vi "FOCUS_V42.vi"(9 "X-pixels":sgl=256.0, 11 "Run":bool) -> (0 "Retrace pixels":sgl, 10 "Pixel Clock (Hz)":sgl)   [LabVIEW 2010] (continued)
                n476 = Add(x=w2193, y="x jog") -> (x+y=w2188:dbl[])
                n477 = And(x=w2107, y=TRUE ("XScale")) -> (x .and. y?=w2106:bool)
                n478 = Delete From Array(array=w2144, length=w2139, index=0) -> (deleted portion=w2142:dbl[], array with subset deleted=w2141:dbl[])
                n479 = Build Array (concatenate)(w2141, w2142) -> (w2111:dbl[])
                n480 = case shown="False" w2109 {
                  tunnel: w2188 -> [w2215 w2219]
                  tunnel: w2184 -> [w2214 w2218]
                  tunnel: [w2213 w2216] -> w2174
                  tunnel: w2111 -> [w2207 w2217]
                  frame False {
                    n481 = local read "Position piezo [µm]"() -> (w2211:sgl)
                    n482 = Multiply(x=sgl 40.0 ("y"), y=w2207) -> (x*y=w2208:dbl[])
                    n483 = Subtract(x=w2208, y=w2211) -> (x-y=w2206:dbl[])
                    n484 = local read "scattering length [µm]"() -> (w2209:sgl)
                    n485 = Divide(x=w2206, y=w2209) -> (x/y=w2205:dbl[])
                    n486 = local read "Intensity"() -> (w2212:sgl)
                    n487 = Exponential(1:w2205) -> (0:w2204:dbl[])
                    n488 = Multiply(x=w2204, y=w2212) -> (x*y=w2203:dbl[])
                    n489 = Build Array(w2215, w2214, w2207, w2203) -> (w2213:dbl[][])
                  }
                  frame True {
                    n490 = Build Array(w2219, w2218, w2217) -> (w2216:dbl[][])
                  }
                }
                n491 = case shown="True" w2109 {
                  tunnel: w2189 -> [_ w2262]
                  tunnel: [w2253 w2255] -> w2187
                  tunnel: [w2254 w2256] -> w2186
                  tunnel: w2174 -> [w2254 w2257]
                  frame False {
                    n492 = local read "total pixels in frame"() -> (w2253:sgl)
                  }
                  frame True {
                    n493 = local read "Scan Block Length"() -> (w2261:sgl)
                    n494 = Multiply(x=w2261, y=w2262) -> (x*y=w2260:sgl)
                    n495 = Multiply(x=w2260, y=1.0) -> (x*y=w2255:dbl)
                    n496 = Initialize Array(0.0 ("element"), 2 ("dimension size"), w2255) -> ()  [unwired: 1 out]
                    n497 = Array Subset(array=w2257, length (col)=w2255) -> (w2256:dbl[][])  [unwired: 3 in]
                  }
                }
                "y scan signals" <- w2168
                "x scan signals" <- w2169
              }
              frame 1 {
                n498 = local read "[µm] per pixel at zoom 1"() -> (w2304:sgl)
                n499 = local read "Y-lines"() -> (w2303:sgl)
                n500 = local read "Rotation z"() -> (w2279:sgl)
                n501 = local read "On?"() -> (w2280:bool)
                n502 = local read "Scanner dead time"() -> (w2296:sgl)
                n503 = case shown="False" w2280 {
                  tunnel: w2279 -> [_ w2419]
                  tunnel: [sgl 0.0 ("Rotation z") w2419] -> w2278
                  frame False {
                  }
                  frame True {
                  }
                }
                n504 = Divide(x=w2278, y=360.0) -> (x/y=w2350:dbl)
                n505 = Multiply(x=w2350, y=6.283185307179586) -> (x*y=w2348:dbl)
                n506 = Build Array(w2354, w2353, w2352) -> (w2334:dbl[][])
                n507 = Divide(x=w2296, y=w2291) -> (x/y=w2298:sgl)
                n508 = Sine(x=w2348) -> (sin(x)=w2307:dbl)
                n509 = Cosine(x=w2348) -> (cos(x)=w2347:dbl)
                n510 = Multiply(x=w2304, y=w2303) -> (x*y=w2301:sgl)
                n511 = Add(x=sgl 2.0, y=w2298) -> (x+y=w2297:sgl)
                n512 = Negate(x=w2307) -> (-x=w2346:dbl)
                n513 = Array Subset(array=w2334, length (row)=1 ("length")) -> (w2337:dbl[][])  [unwired: 3 in]
                n514 = Array Subset(array=w2334, index (row)=1 ("index")) -> (w2341:dbl[][])  [unwired: 3 in]
                n515 = local read "Zoom"() -> (w2308:sgl)
                n516 = Build Array(w2307, w2347) -> (w2343:dbl[])
                n517 = Build Array(w2347, w2346) -> (w2344:dbl[])
                n518 = local read "total y pixels"() -> (w2293:sgl)
                n519 = Round To Nearest(number=w2297) -> (nearest integer value=w2295:sgl)
                n520 = Build Array(w2344, w2343) -> (w2342:dbl[][])
                n521 = local read "Rotation"() -> (w2358:sgl)
                n522 = call-poly <vilib>:"A x B.vi"("B"=w2341, "A"=w2342) -> ("A x B"=w2335:T15)  [unwired: 1 out]
                n523 = local read "Position piezo [µm]"() -> (w2306:sgl)
                n524 = Divide(x=w2301, y=w2308) -> (x/y=w2312:sgl)
                n525 = local read "x-step (um)"() -> (w2285:sgl)
                n526 = local read "y-step (um)"() -> (w2286:sgl)
                n527 = local read "z-step (um)"() -> (w2300:sgl)
                n528 = local read "total x pixels"() -> (w2294:sgl)
                n529 = Divide(x=w2312, y=sgl 40.0) -> (x/y=w2318:sgl)
                n530 = Multiply(x=w2358, y=-1.0) -> (x*y=w2361:dbl)
                n531 = Index Array(array=w2335, index (row)=0 ("disabled index (col)")) -> (element=w2336:dbl[])  [unwired: 1 in]
                n532 = Index Array(array=w2335, index (row)=1 ("disabled index (col)")) -> (element=w2309:dbl[])  [unwired: 1 in]
                n533 = Array Max & Min(array=w2309) -> (max value=w2310:dbl, min value=w2315:dbl)  [unwired: 2 out]
                n534 = Subtract(x=w2310, y=w2315) -> (x-y=w2317:dbl)
                n535 = local read "Mode selector"() -> (w2272:u16)
                n536 = Equal To 0?(x=w2317) -> (x = 0?=w2320:bool)
                n537 = Subtract(x=w2309, y=w2315) -> (x-y=w2321:dbl[])
                n538 = Subtract(x=w2361, y=360.0) -> (x-y=w2359:dbl)
                n539 = Multiply(x=w2318, y=w2307) -> (x*y=w2319:dbl)
                n540 = Divide(x=w2359, y=360.0) -> (x/y=w2367:dbl)
                n541 = Build Array (concatenate)(w2337, w2336) -> (w2333:dbl[][])
                n542 = Equal To 0?(x=w2285) -> (x = 0?=w2284:bool)
                n543 = Equal To 0?(x=w2286) -> (x = 0?=w2283:bool)
                n544 = Equal To 0?(x=w2300) -> (x = 0?=w2282:bool)
                n545 = Divide(x=w2306, y=sgl 40.0) -> (x/y=w2302:sgl)
                n546 = case shown="False" w2320 {
                  tunnel: [w2447 w2448] -> w2316
                  tunnel: w2317 -> [w2446 _]
                  tunnel: w2319 -> [w2444 _]
                  tunnel: w2302 -> [w2442 w2450]
                  tunnel: w2321 -> [w2436 w2449]
                  frame False {
                    n547 = Divide(x=w2436, y=w2446) -> (x/y=w2445:dbl[])
                    n548 = Multiply(x=w2445, y=w2444) -> (x*y=w2443:dbl[])
                    n549 = Add(x=w2443, y=w2442) -> (x+y=w2435:dbl[])
                    n550 = Array Max & Min(array=w2435) -> (max value=w2441:dbl, min value=w2438:dbl)  [unwired: 2 out]
                    n551 = Subtract(x=w2441, y=w2438) -> (x-y=w2440:dbl)
                    n552 = Divide(x=w2440, y=2.0) -> (x/y=w2437:dbl)
                    n553 = Subtract(x=w2435, y=w2437) -> (x-y=w2447:dbl[])
                  }
                  frame True {
                    n554 = Add(x=w2449, y=w2450) -> (x+y=w2448:dbl[])
                  }
                }
                n555 = Multiply(x=w2367, y=6.283185307179586) -> (x*y=w2369:dbl)
                n556 = Compound Arithmetic op=AND(w2284, w2283, w2282) -> (w2281:bool)
                n557 = Equal?(x=w2272, y=u16 4) -> (x = y?=w2265:bool)
                n558 = Sine(x=w2369) -> (sin(x)=w2373:dbl)
                n559 = Cosine(x=w2369) -> (cos(x)=w2374:dbl)
                n560 = case shown="False" w2281 {
                  tunnel: [w2427 w2434] -> w2292
                  tunnel: w2295 -> [w2422 w2430]
                  frame True {
                    w2426 = 10178 items=["Finite Samples"=10178, "Continuous Samples"=10123, "Hardware Timed Single Point"=12522] ("sample mode")
                    n561 = local read "total pixels in frame"() -> (w2424:sgl)
                    n562 = local read "Number of frames"() -> (w2423:sgl)
                    n563 = local read "Averaging"() -> (w2425:u16)
                    n564 = Compound Arithmetic op=MULTIPLY(w2425, w2423, w2424) -> (w2421:sgl)
                    n565 = Add(x=w2421, y=w2422) -> (x+y=w2420:sgl)
                    n566 = Bundle(w2420, "sample mode"=w2426) -> (w2427:cluster{sgl, "sample mode":i32})  [unwired: 1 in]
                  }
                  frame False {
                    w2433 = 10178 items=["Finite Samples"=10178, "Continuous Samples"=10123, "Hardware Timed Single Point"=12522] ("sample mode")
                    n567 = local read "total pixels in frame"() -> (w2431:sgl)
                    n568 = local read "Averaging"() -> (w2432:u16)
                    n569 = Compound Arithmetic op=MULTIPLY(w2432, w2431) -> (w2429:sgl)
                    n570 = Add(x=w2429, y=w2430) -> (x+y=w2428:sgl)
                    n571 = Bundle(w2428, "sample mode"=w2433) -> (w2434:cluster{sgl, "sample mode":i32})  [unwired: 1 in]
                  }
                }
                n572 = Negate(x=w2373) -> (-x=w2370:dbl)
                n573 = local read "FocusModeSelector"() -> (w2276:bool)
                n574 = Build Array(w2374, w2370) -> (w2371:dbl[])
                n575 = Build Array(w2373, w2374) -> (w2372:dbl[])
                n576 = Build Array(w2371, w2372) -> (w2357:dbl[][])
                n577 = call-poly <vilib>:"A x B.vi"("B"=w2333, "A"=w2357) -> ("A x B"=w2332:T15)  [unwired: 1 out]
                n578 = In Range and Coerce(upper limit=0.0 ("element"), x=w2316, lower limit=10.0 ("element")) -> (coerced(x)=w2329:dbl[])  [unwired: 1 out]
                n579 = Divide(x=w2332, y=w2308) -> (x/y=w2331:T15)
                n580 = Array Size(array=w2329) -> (size(s)=w2328:i32)
                n581 = local read "x jog"() -> (w2289:sgl)
                n582 = local read "y jog"() -> (w2288:sgl)
                n583 = case shown="True" w2276 {
                  tunnel: w2267 -> [w2409 w2417]
                  tunnel: [w2408 w2416] -> w2266
                  tunnel: w2268 -> [w2407 w2415]
                  frame True {
                    n584 = Concatenate Strings(w2407, tag "/ao0," ("physical channels"), w2407, tag "/ao1," ("physical channels"), w2407, tag "/ao2" ("physical channels")) -> (w2404:string)
                    n585 = Type Cast(type=w2409, x=w2404) -> (*(type *) &x=w2408:tag)
                  }
                  frame False {
                    n586 = Concatenate Strings(w2415, tag "/ao0," ("physical channels"), w2415, tag "/ao1," ("physical channels"), w2415, tag "/ao2," ("physical channels"), w2415, tag "/ao3" ("physical channels")) -> (w2412:string)
                    n587 = Type Cast(type=w2417, x=w2412) -> (*(type *) &x=w2416:tag)
                  }
                }
                n588 = case shown="True" w2265 {
                  tunnel: w2267 -> [w2380 _]
                  tunnel: [w2379 w2381] -> w2264
                  tunnel: w2268 -> [w2378 _]
                  tunnel: w2266 -> [_ w2381]
                  frame True {
                    n589 = Concatenate Strings(w2378, tag "/ao0," ("physical channels"), w2378, tag "/ao1" ("physical channels")) -> (w2375:string)
                    n590 = Type Cast(type=w2380, x=w2375) -> (*(type *) &x=w2379:tag)
                  }
                  frame False {
                  }
                }
                n591 = Index Array(array=w2331, index (row)=0 ("disabled index (col)")) -> (element=w2365:dbl[])  [unwired: 1 in]
                n592 = Index Array(array=w2331, index (row)=1 ("disabled index (col)")) -> (element=w2364:dbl[])  [unwired: 1 in]
                n593 = Multiply(x=w2328, y=15) -> (x*y=w2323:i32)
                n594 = local read "total pixels in frame"() -> (w2290:sgl)
                n595 = Divide(x=w2323, y=360.0) -> (x/y=w2324:dbl)
                n596 = Add(x=w2364, y=w2288) -> (x+y=w2273:dbl[])
                n597 = Add(x=w2365, y=w2289) -> (x+y=w2274:dbl[])
                n598 = Not(x=w2276) -> (.not. x?=w2275:bool)
                n599 = Delete From Array(array=w2329, length=w2324, index=0) -> (deleted portion=w2327:dbl[], array with subset deleted=w2326:dbl[])
                n600 = Build Array (concatenate)(w2326, w2327) -> (w2277:dbl[])
                n601 = case shown="False" w2276 {
                  tunnel: w2274 -> [w2398 w2402]
                  tunnel: w2273 -> [w2397 w2401]
                  tunnel: [w2396 w2399] -> w2270
                  tunnel: w2277 -> [w2393 w2400]
                  frame False {
                    n602 = local read "Position piezo [µm]"() -> (w2388:sgl)
                    n603 = Multiply(x=sgl 40.0 ("y"), y=w2393) -> (x*y=w2394:dbl[])
                    n604 = Subtract(x=w2394, y=w2388) -> (x-y=w2392:dbl[])
                    n605 = local read "scattering length [µm]"() -> (w2387:sgl)
                    n606 = Divide(x=w2392, y=w2387) -> (x/y=w2391:dbl[])
                    n607 = Exponential(1:w2391) -> (0:w2390:dbl[])
                    n608 = local read "Intensity"() -> (w2386:sgl)
                    n609 = Multiply(x=w2390, y=w2386) -> (x*y=w2389:dbl[])
                    n610 = Build Array(w2398, w2397, w2393, w2389) -> (w2396:dbl[][])
                  }
                  frame True {
                    n611 = Build Array(w2402, w2401, w2400) -> (w2399:dbl[][])
                  }
                }
                n612 = case shown="False" w2265 {
                  tunnel: w2274 -> [_ w2385]
                  tunnel: w2273 -> [_ w2384]
                  tunnel: w2270 -> [w2382 _]
                  tunnel: [w2382 w2383] -> w2269
                  frame False {
                  }
                  frame True {
                    n613 = Build Array(w2385, w2384) -> (w2383:dbl[][])
                  }
                }
              }
              frame 2 {
                w2465 = 10123 items=["Finite Samples"=10178, "Continuous Samples"=10123, "Hardware Timed Single Point"=12522] ("sample mode")
                n614 = local read "[µm] per pixel at zoom 1"() -> (w2472:sgl)
                n615 = local read "Y-lines"() -> (w2471:sgl)
                n616 = local read "Rotation z"() -> (w2452:sgl)
                n617 = local read "On?"() -> (w2453:bool)
                n618 = case shown="False" w2453 {
                  tunnel: w2452 -> [_ w2552]
                  tunnel: [sgl 0.0 ("Rotation z") w2552] -> w2451
                  frame False {
                  }
                  frame True {
                  }
                }
                n619 = Divide(x=w2451, y=360.0) -> (x/y=w2519:dbl)
                n620 = case shown="False" "Linescan mode" {
                  tunnel: w2458 -> [w2554 _]
                  tunnel: [w2554 w2557] -> w2457
                  tunnel: [w2553 w2558] -> w2456
                  tunnel: w2455 -> [_ w2558]
                  frame False {
                    n621 = Array Size(array=w2554) -> (size(s)=w2555:i32)
                    n622 = Initialize Array(0.0 ("element"), w2555) -> (w2553:dbl[])
                  }
                  frame True {
                    n623 = Array Size(array=w2558) -> (size(s)=w2559:i32)
                    n624 = Initialize Array(0.0 ("element"), w2559) -> (w2557:dbl[])
                  }
                }
                n625 = Multiply(x=w2519, y=6.283185307179586) -> (x*y=w2517:dbl)
                n626 = Build Array(w2457, w2456, w2521) -> (w2503:dbl[][])
                n627 = Sine(x=w2517) -> (sin(x)=w2475:dbl)
                n628 = Cosine(x=w2517) -> (cos(x)=w2516:dbl)
                n629 = Multiply(x=w2472, y=w2471) -> (x*y=w2469:sgl)
                n630 = Negate(x=w2475) -> (-x=w2515:dbl)
                n631 = Array Subset(array=w2503, length (row)=1 ("length")) -> (w2506:dbl[][])  [unwired: 3 in]
                n632 = Array Subset(array=w2503, index (row)=1 ("index")) -> (w2510:dbl[][])  [unwired: 3 in]
                n633 = local read "Zoom"() -> (w2477:sgl)
                n634 = Build Array(w2475, w2516) -> (w2512:dbl[])
                n635 = Build Array(w2516, w2515) -> (w2513:dbl[])
                n636 = local read "total y pixels"() -> (w2463:sgl)
                n637 = Build Array(w2513, w2512) -> (w2511:dbl[][])
                n638 = local read "Rotation"() -> (w2532:sgl)
                n639 = local read "total x pixels"() -> (w2462:sgl)
                n640 = call-poly <vilib>:"A x B.vi"("B"=w2510, "A"=w2511) -> ("A x B"=w2504:T15)  [unwired: 1 out]
                n641 = local read "Position piezo [µm]"() -> (w2474:sgl)
                n642 = Divide(x=w2469, y=w2477) -> (x/y=w2481:sgl)
                n643 = Divide(x=w2481, y=sgl 40.0) -> (x/y=w2487:sgl)
                n644 = Multiply(x=w2532, y=-1.0) -> (x*y=w2535:dbl)
                n645 = Index Array(array=w2504, index (row)=0 ("disabled index (col)")) -> (element=w2505:dbl[])  [unwired: 1 in]
                n646 = Index Array(array=w2504, index (row)=1 ("disabled index (col)")) -> (element=w2478:dbl[])  [unwired: 1 in]
                n647 = Array Max & Min(array=w2478) -> (max value=w2479:dbl, min value=w2484:dbl)  [unwired: 2 out]
                n648 = Subtract(x=w2479, y=w2484) -> (x-y=w2486:dbl)
                n649 = Equal To 0?(x=w2486) -> (x = 0?=w2489:bool)
                n650 = Subtract(x=w2478, y=w2484) -> (x-y=w2490:dbl[])
                n651 = Subtract(x=w2535, y=360.0) -> (x-y=w2533:dbl)
                n652 = Multiply(x=w2487, y=w2475) -> (x*y=w2488:dbl)
                n653 = Divide(x=w2533, y=360.0) -> (x/y=w2543:dbl)
                n654 = Build Array (concatenate)(w2506, w2505) -> (w2502:dbl[][])
                n655 = Divide(x=w2474, y=sgl 40.0) -> (x/y=w2470:sgl)
                n656 = case shown="False" w2489 {
                  tunnel: [w2573 w2574] -> w2485
                  tunnel: w2486 -> [w2572 _]
                  tunnel: w2488 -> [w2570 _]
                  tunnel: w2470 -> [w2568 w2576]
                  tunnel: w2490 -> [w2562 w2575]
                  frame False {
                    n657 = Divide(x=w2562, y=w2572) -> (x/y=w2571:dbl[])
                    n658 = Multiply(x=w2571, y=w2570) -> (x*y=w2569:dbl[])
                    n659 = Add(x=w2569, y=w2568) -> (x+y=w2561:dbl[])
                    n660 = Array Max & Min(array=w2561) -> (max value=w2567:dbl, min value=w2564:dbl)  [unwired: 2 out]
                    n661 = Subtract(x=w2567, y=w2564) -> (x-y=w2566:dbl)
                    n662 = Divide(x=w2566, y=2.0) -> (x/y=w2563:dbl)
                    n663 = Subtract(x=w2561, y=w2563) -> (x-y=w2573:dbl[])
                  }
                  frame True {
                    n664 = Add(x=w2575, y=w2576) -> (x+y=w2574:dbl[])
                  }
                }
                n665 = Multiply(x=w2543, y=6.283185307179586) -> (x*y=w2545:dbl)
                n666 = Sine(x=w2545) -> (sin(x)=w2549:dbl)
                n667 = Cosine(x=w2545) -> (cos(x)=w2550:dbl)
                n668 = Negate(x=w2549) -> (-x=w2546:dbl)
                n669 = Build Array(w2550, w2546) -> (w2547:dbl[])
                n670 = Build Array(w2549, w2550) -> (w2548:dbl[])
                n671 = Bundle("sample mode"=w2465, "sample mode"=w2465) -> (w2461:cluster{"sample mode":i32, "sample mode":i32})  [unwired: 1 in]
                n672 = Build Array(w2547, w2548) -> (w2531:dbl[][])
                n673 = call-poly <vilib>:"A x B.vi"("B"=w2502, "A"=w2531) -> ("A x B"=w2501:T15)  [unwired: 1 out]
                n674 = In Range and Coerce(upper limit=0.0 ("element"), x=w2485, lower limit=10.0 ("element")) -> (coerced(x)=w2498:dbl[])  [unwired: 1 out]
                n675 = Divide(x=w2501, y=w2477) -> (x/y=w2500:T15)
                n676 = Array Size(array=w2498) -> (size(s)=w2497:i32)
                n677 = local read "x jog"() -> (w2467:sgl)
                n678 = local read "y jog"() -> (w2466:sgl)
                n679 = Index Array(array=w2500, index (row)=0 ("disabled index (col)")) -> (element=w2541:dbl[])  [unwired: 1 in]
                n680 = Index Array(array=w2500, index (row)=1 ("disabled index (col)")) -> (element=w2540:dbl[])  [unwired: 1 in]
                n681 = Multiply(x=w2497, y=15) -> (x*y=w2492:i32)
                n682 = Divide(x=w2492, y=360.0) -> (x/y=w2493:dbl)
                n683 = Add(x=w2540, y=w2466) -> (x+y=w2537:dbl[])
                n684 = Multiply(x=w2462, y=sgl 1.0) -> (x*y=w2460:sgl)
                n685 = Add(x=w2541, y=w2467) -> (x+y=w2539:dbl[])
                n686 = Delete From Array(array=w2498, length=w2493, index=0) -> (deleted portion=w2496:dbl[], array with subset deleted=w2495:dbl[])
                n687 = Concatenate Strings(w2527, tag "/ao0," ("physical channels"), w2527, tag "/ao1," ("physical channels"), w2527, tag "/ao2" ("physical channels")) -> (w2523:string)
                n688 = Build Array (concatenate)(w2495, w2496) -> (w2476:dbl[])
                n689 = Build Array(w2539, w2537, w2476) -> (w2468:dbl[][])
                n690 = Type Cast(type=w2528, x=w2523) -> (*(type *) &x=w2526:tag)
              }
              frame 3 {
                w2581 = 10123 items=["Finite Samples"=10178, "Continuous Samples"=10123, "Hardware Timed Single Point"=12522] ("sample mode")
                n691 = case shown="True" w2591 {
                  tunnel: w2595 -> [_ _]
                  tunnel: [w2599 w2618] -> w2590
                  tunnel: [w2601 w2636] -> w2594
                  tunnel: [w2600 w2613] -> w2593
                  tunnel: [w2600 w2613] -> w2592
                  tunnel: w2579 -> [_ w2610]
                  tunnel: w2578 -> [_ w2606]
                  frame False {
                    n692 = local read "Y-lines FreeLine"() -> (w2601:sgl)
                    n693 = local read "X-pixels FreeLine"() -> (w2600:sgl)
                    n694 = local read "y scan signals"() -> (w2596:dbl[])
                    n695 = Array Max & Min(array=w2596) -> (max value=w2598:dbl, min value=w2597:dbl)  [unwired: 2 out]
                    n696 = property on="XY Graph 1" class="XYGraph (strict)"("X Scale.Range:Maximum"=w2598, "X Scale.Range:Minimum"=w2597, "Y Scale.Range:Maximum"=w2598, "Y Scale.Range:Minimum"=w2597) -> ()  [unwired: 2 in, 2 out]
                    n697 = property on="XY Graph 2" class="XYGraph (strict)"("X Scale.Range:Maximum"=w2598, "X Scale.Range:Minimum"=w2597, "Y Scale.Range:Maximum"=w2598, "Y Scale.Range:Minimum"=w2597) -> ()  [unwired: 2 in, 2 out]
                    n698 = local read "ScanLineFreeLine"() -> (w2599:sgl[][])
                  }
                  frame True {
                    w2654 = 1 ("length")
                    # "Rotation"
                    n699 = local read "Scan Cut-Off (either end)"() -> (w2603:sgl)
                    n700 = Index Array(array=w2606, index=w2603) -> (element=w2609:dbl)
                    n701 = local read "X-pixels"() -> (w2605:sgl)
                    n702 = local read "Y-lines"() -> (w2604:sgl)
                    n703 = property on="XY Graph 2" class="XYGraph (strict)"("Visible"=TRUE) -> ()  [unwired: 2 in, 2 out]
                    n704 = property on="XY Graph 1" class="XYGraph (strict)"("Visible"=TRUE) -> ()  [unwired: 2 in, 2 out]
                    n705 = Divide(x=w2605, y=w2604) -> (x/y=w2608:sgl)
                    n706 = property on="Image 2" class="IntGraph (strict)"() -> ("Color Table"=w2644:u32[])  [unwired: 2 in, 2 out]
                    n707 = Divide(x=w2609, y=w2608) -> (x/y=w2607:dbl)
                    n708 = Absolute Value(x=w2607) -> (abs(x)=w2602:dbl)
                    n709 = local read "Image 2"() -> (w2669:u8[][])
                    n710 = local read "Image 1"() -> (w2668:u8[][])
                    n711 = local read "X-pixels"() -> (w2633:sgl)
                    n712 = local read "Y-lines"() -> (w2632:sgl)
                    n713 = call "FreeLine2D.vi"("Color Table"=w2644, "data channel 2"=w2669, "X-pixels"=w2633, "Y-lines"=w2632, "data channel"=w2668) -> ("user defined lines"=w2636:i16, "PointsCoordinates"=w2638:i32[][], "pixel x"=w2635:dbl[], "pixel y"=w2634:dbl[], "number of pixels"=w2613:dbl, "Pixel Clock (Hz)"=w2612:dbl)
                    "X-pixels FreeLine" <- w2613
                    "Pixel Clock (Hz) FreeLine" <- w2612
                    n714 = local write "Y-lines FreeLine"(w2636) -> ()
                    n715 = Array Max & Min(array=w2610) -> (max value=w2617:dbl, min value=w2616:dbl)  [unwired: 2 out]
                    n716 = call "CalcxyscansignalsudlFOCUS.vi"("Y-Lines"=w2632, "X Pixels"=w2633, "MaxValuey"=w2602, "MaxValuex"=w2602, "pixel y"=w2634, "pixel x"=w2635) -> ("Signal y"=w2630:dbl[], "Signal x"=w2631:dbl[])
                    n717 = Index Array(array=w2638, index (col)=0 ("disabled index (col)")) -> (element=w2642:i32[])  [unwired: 1 in]
                    n718 = Index Array(array=w2638, index (col)=1 ("disabled index (col)")) -> (element=w2641:i32[])  [unwired: 1 in]
                    n719 = local write "new FreeLine?"(FALSE ("new udl?")) -> ()
                    n720 = Bundle("PointsCoordinates"=w2642, "PointsCoordinates"=w2641) -> (w2637:T16)  [unwired: 1 in]
                    n721 = local read "Rotation"() -> (w2626:sgl)
                    n722 = property on="XY Graph 1" class="XYGraph (strict)"("X Scale.Range:Maximum"=w2617, "X Scale.Range:Minimum"=w2616, "Y Scale.Range:Maximum"=w2617, "Y Scale.Range:Minimum"=w2616) -> ()  [unwired: 2 in, 2 out]
                    n723 = Build Array(w2631, w2630) -> (w2623:dbl[][])
                    n724 = Multiply(x=w2626, y=-1.0) -> (x*y=w2628:dbl)
                    n725 = local write "Histogram1"(w2637) -> ()
                    n726 = local write "Histogram2"(w2637) -> ()
                    n727 = Subtract(x=w2628, y=360.0) -> (x-y=w2625:dbl)
                    n728 = local read "Zoom"() -> (w2651:sgl)
                    n729 = Divide(x=w2625, y=360.0) -> (x/y=w2677:dbl)
                    n730 = property on="XY Graph 2" class="XYGraph (strict)"("X Scale.Range:Maximum"=w2617, "X Scale.Range:Minimum"=w2616, "Y Scale.Range:Maximum"=w2617, "Y Scale.Range:Minimum"=w2616) -> ()  [unwired: 2 in, 2 out]
                    n731 = Multiply(x=w2677, y=6.283185307179586) -> (x*y=w2675:dbl)
                    n732 = Divide(x=w2623, y=w2651) -> (x/y=w2622:dbl[][])
                    n733 = Reciprocal(x=w2612) -> (1/x=w2615:dbl)
                    n734 = property on="XY Graph 3" class="XYGraph (strict)"("X Scale.Range:Maximum"=w2617, "X Scale.Range:Minimum"=w2616, "Y Scale.Range:Maximum"=w2617, "Y Scale.Range:Minimum"=w2616) -> ()  [unwired: 2 in, 2 out]
                    n735 = Sine(x=w2675) -> (sin(x)=w2671:dbl)
                    n736 = Cosine(x=w2675) -> (cos(x)=w2670:dbl)
                    n737 = Negate(x=w2671) -> (-x=w2674:dbl)
                    n738 = Multiply(x=w2615, y=sgl 1000000.0) -> (x*y=w2611:dbl)
                    n739 = Array Subset(array=w2631, index=0, length=1) -> (w2661:dbl[])
                    n740 = Array Subset(array=w2630, index=0, length=1) -> (w2660:dbl[])
                    n741 = local write "pixel dwell time [us] FreeLine"(w2611) -> ()
                    n742 = Build Array(w2670, w2674) -> (w2673:dbl[])
                    n743 = Build Array(w2671, w2670) -> (w2672:dbl[])
                    n744 = property on="XY Graph 4" class="XYGraph (strict)"("X Scale.Range:Maximum"=w2617, "X Scale.Range:Minimum"=w2616, "Y Scale.Range:Maximum"=w2617, "Y Scale.Range:Minimum"=w2616) -> ()  [unwired: 2 in, 2 out]
                    n745 = Bundle("Signal x"=w2631, "Signal y"=w2630) -> (w2659:cluster{"Signal x":dbl[], "Signal y":dbl[]})  [unwired: 1 in]
                    n746 = Bundle(w2661, w2660) -> (w2658:cluster{dbl[], dbl[]})  [unwired: 1 in]
                    n747 = Build Array(w2673, w2672) -> (w2624:dbl[][])
                    n748 = Decrement(x=w2613) -> (x-1=w2653:dbl)
                    n749 = Array Subset(array=w2631, index=w2653, length=w2654) -> (w2655:dbl[])
                    n750 = Array Subset(array=w2630, index=w2653, length=w2654) -> (w2656:dbl[])
                    n751 = call-poly <vilib>:"A x B.vi"("B"=w2622, "A"=w2624) -> ("A x B"=w2621:T15)  [unwired: 1 out]
                    n752 = Bundle(w2655, w2656) -> (w2652:cluster{dbl[], dbl[]})  [unwired: 1 in]
                    n753 = local read "x jog"() -> (w2645:sgl)
                    n754 = Index Array(array=w2621, index (row)=0 ("disabled index (col)")) -> (element=w2650:dbl[])  [unwired: 1 in]
                    n755 = Index Array(array=w2621, index (row)=1 ("disabled index (col)")) -> (element=w2649:dbl[])  [unwired: 1 in]
                    n756 = Build Array(w2659, w2658, w2652) -> (→"XY Graph 1" →"XY Graph 2":cluster{"Signal x":dbl[], "Signal y":dbl[]}[])
                    n757 = local read "y jog"() -> (w2646:sgl)
                    n758 = Add(x=w2649, y=w2646) -> (x+y=w2647:dbl[])
                    n759 = Add(x=w2650, y=w2645) -> (x+y=w2648:dbl[])
                    n760 = Build Array(w2648, w2647) -> (w2618:dbl[][])
                    "ScanLineFreeLine" <- w2618
                  }
                }
                n761 = Bundle("sample mode"=w2581, "sample mode"=w2581) -> (w2580:cluster{"sample mode":i32, "sample mode":i32})  [unwired: 1 in]
                n762 = local write "XScale"(TRUE ("XScale")) -> ()
                n763 = Concatenate Strings(w2585, tag "/ao0," ("physical channels"), w2585, tag "/ao1" ("physical channels")) -> (w2587:string)
                n764 = Type Cast(type=w2584, x=w2587) -> (*(type *) &x=w2583:tag)
              }
              frame 4 {
                w2685 = 10123 items=["Finite Samples"=10178, "Continuous Samples"=10123, "Hardware Timed Single Point"=12522] ("sample mode")
                n765 = case shown="True" w2694 {
                  tunnel: [w2730 w2782] -> w2700
                  tunnel: [w2729 w2745] -> w2696
                  tunnel: w2699 -> [_ _]
                  tunnel: [w2705 w2754] -> w2698
                  tunnel: [w2729 w2745] -> w2697
                  tunnel: w2683 -> [_ w2748]
                  tunnel: w2682 -> [_ w2747]
                  tunnel: w2681 -> [_ w2738]
                  tunnel: w2680 -> [_ w2737]
                  frame False {
                    n766 = local read "Zsin3D"() -> (w2713:sgl[])
                    n767 = local read "Amplitude Factor"() -> (w2711:sgl)
                    n768 = local read "y scan signals"() -> (w2719:dbl[])
                    n769 = Array Size(array=w2713) -> (size(s)=w2718:i32)
                    n770 = Add Array Elements(numeric array=w2713) -> (sum=w2717:sgl)
                    n771 = Divide(x=w2717, y=w2718) -> (x/y=w2714:sgl)
                    n772 = Subtract(x=w2713, y=w2714) -> (x-y=w2716:sgl[])
                    n773 = Multiply(x=w2716, y=w2711) -> (x*y=w2715:sgl[])
                    n774 = local read "phase shift [°]"() -> (w2722:sgl)
                    n775 = Array Max & Min(array=w2719) -> (max value=w2721:dbl, min value=w2720:dbl)  [unwired: 2 out]
                    n776 = Add(x=w2715, y=w2714) -> (x+y=w2712:sgl[])
                    n777 = local read "Y-lines FreeLine"() -> (w2730:sgl)
                    n778 = local read "X-pixels FreeLine"() -> (w2729:sgl)
                    n779 = property on="XY Graph 1" class="XYGraph (strict)"("X Scale.Range:Maximum"=w2721, "X Scale.Range:Minimum"=w2720, "Y Scale.Range:Maximum"=w2721, "Y Scale.Range:Minimum"=w2720) -> ()  [unwired: 2 in, 2 out]
                    n780 = Array Size(array=w2712) -> (size(s)=w2706:i32)
                    n781 = Multiply(x=w2706, y=w2722) -> (x*y=w2727:sgl)
                    n782 = Divide(x=w2727, y=360.0) -> (x/y=w2726:dbl)
                    n783 = property on="XY Graph 2" class="XYGraph (strict)"("X Scale.Range:Maximum"=w2721, "X Scale.Range:Minimum"=w2720, "Y Scale.Range:Maximum"=w2721, "Y Scale.Range:Minimum"=w2720) -> ()  [unwired: 2 in, 2 out]
                    n784 = local read "Intensity"() -> (w2707:sgl)
                    n785 = local read "ZInt3D"() -> (w2708:sgl[])
                    n786 = Delete From Array(array=w2712, length=w2726, index=0) -> (deleted portion=w2723:sgl[], array with subset deleted=w2724:sgl[])
                    n787 = Build Array (concatenate)(w2724, w2723) -> (w2710:sgl[])
                    n788 = Multiply(x=w2708, y=w2707) -> (x*y=w2702:sgl[])
                    n789 = Initialize Array(w2707, w2706) -> ()  [unwired: 1 out]
                    n790 = property on="Histogram1" class="XYGraph (strict)"("Visible"=FALSE) -> ()  [unwired: 2 in, 2 out]
                    n791 = case shown="True" "Int Corr?" {
                      tunnel: w2702 -> [w2731 w2736]
                      tunnel: [w2731 w2735] -> w2701
                      frame False {
                      }
                      frame True {
                        n792 = local read "Image3Arrayd"() -> (w2732:u8[][])
                        n793 = call "NormalizeIntensityUDL3D.vi"("bigger"="Scale", "Image3Array"=w2732, "Pockel's cell original"=w2736, "File?"=FALSE) -> ("Pockel's cell corrected"=w2735:dbl[])
                      }
                    }
                    n794 = local read "ScanLineFreeLine"() -> (w2709:sgl[][])
                    n795 = Build Array (concatenate)(w2709, w2710, w2701) -> (w2705:dbl[][])
                  }
                  frame True {
                    w2820 = 1 ("length")
                    # "Rotation"
                    n796 = property on="Image 2" class="IntGraph (strict)"() -> ("Color Table"=w2791:u32[])  [unwired: 2 in, 2 out]
                    n797 = local read "Scan Cut-Off (either end)"() -> (w2800:sgl)
                    n798 = local write "new FreeLine?"(FALSE ("new 3D udl?")) -> ()
                    n799 = local read "pixelstoµm"() -> (w2812:sgl)
                    n800 = property on="XY Graph 2" class="XYGraph (strict)"("Visible"=TRUE) -> ()  [unwired: 2 in, 2 out]
                    n801 = property on="XY Graph 1" class="XYGraph (strict)"("Visible"=TRUE) -> ()  [unwired: 2 in, 2 out]
                    n802 = local read "Number of frames"() -> (w2816:sgl)
                    n803 = local read "X-pixels"() -> (w2802:sgl)
                    n804 = local read "Y-lines"() -> (w2801:sgl)
                    n805 = Index Array(array=w2738, index=w2800) -> (element=w2739:dbl)
                    n806 = Divide(x=w2802, y=w2801) -> (x/y=w2803:sgl)
                    n807 = local read "X-pixels"() -> (w2770:sgl)
                    n808 = local read "Y-lines"() -> (w2769:sgl)
                    n809 = Divide(x=w2739, y=w2803) -> (x/y=w2799:dbl)
                    n810 = local read "z-step (um)"() -> (w2817:sgl)
                    n811 = Absolute Value(x=w2799) -> (abs(x)=w2771:dbl)
                    n812 = local read "Zoom"() -> (w2813:sgl)
                    n813 = call "FreeLine3D.vi"("Data1"=w2748, "z step (µm)"=w2817, "Color Table"=w2791, "Y-lines"=w2769, "X-pixels"=w2770, "Data2"=w2747, "pixelstoµm"=w2812, "z planes"=w2816, "zoom"=w2813) -> ("user defined lines"=w2782:i16, "x-values [pixels]"=w2773:dbl[], "pockel's cell"=w2752:dbl[], "y-values [pixels]"=w2772:dbl[], "PointsCoordinates"=w2787:i32[][], "pixel clock [Hz]"=w2743:dbl, "z-values [µm]"=w2746:dbl[])
                    "Pixel Clock z (Hz) FreeLine" <- w2743
                    "PointsCoordinates" <- w2787
                    "ZInt3D" <- w2752
                    n814 = local write "Y-lines FreeLine"(w2782) -> ()
                    n815 = Divide(x=w2746, y=40.0) -> (x/y=w2778:dbl[])
                    "Zsin3D" <- w2778
                    n816 = Array Size(array=w2778) -> (size(s)=w2749:i32)
                    n817 = Add Array Elements(numeric array=w2778) -> (sum=w2781:dbl)
                    n818 = Divide(x=w2781, y=w2749) -> (x/y=w2776:dbl)
                    n819 = Subtract(x=w2778, y=w2776) -> (x-y=w2780:dbl[])
                    n820 = Multiply(x=w2780, y="Amplitude Factor") -> (x*y=w2777:dbl[])
                    n821 = Add(x=w2777, y=w2776) -> (x+y=w2775:dbl[])
                    n822 = Array Size(array=w2775) -> (size(s)=w2809:i32)
                    n823 = Array Size(array=w2746) -> (size(s)=w2745:i32)
                    n824 = Array Max & Min(array=w2737) -> (max value=w2790:dbl, min value=w2789:dbl)  [unwired: 2 out]
                    n825 = call "CalcxyscansignalsudlFOCUS.vi"("Y-Lines"=w2769, "X Pixels"=w2770, "MaxValuey"=w2771, "MaxValuex"=w2771, "pixel y"=w2772, "pixel x"=w2773) -> ("Signal y"=w2767:dbl[], "Signal x"=w2768:dbl[])
                    n826 = Multiply(x=w2809, y="phase shift [°]") -> (x*y=w2810:sgl)
                    n827 = Divide(x=w2810, y=360.0) -> (x/y=w2807:dbl)
                    n828 = local write "Pixel Clock (Hz) FreeLine"(w2743) -> ()
                    n829 = Delete From Array(array=w2775, length=w2807, index=0) -> (deleted portion=w2804:dbl[], array with subset deleted=w2805:dbl[])
                    n830 = Build Array(w2768, w2767) -> (w2760:dbl[][])
                    n831 = property on="XY Graph 1" class="XYGraph (strict)"("X Scale.Range:Maximum"=w2790, "X Scale.Range:Minimum"=w2789, "Y Scale.Range:Maximum"=w2790, "Y Scale.Range:Minimum"=w2789) -> ()  [unwired: 2 in, 2 out]
                    n832 = Build Array (concatenate)(w2805, w2804) -> (w2755:dbl[])
                    n833 = Index Array(array=w2787, index (col)=0 ("disabled index (col)")) -> (element=w2788:i32[])  [unwired: 1 in]
                    n834 = Index Array(array=w2787, index (col)=1 ("disabled index (col)")) -> (element=w2786:i32[])  [unwired: 1 in]
                    n835 = local read "Rotation"() -> (w2763:sgl)
                    n836 = local read "Intensity"() -> (w2751:sgl)
                    n837 = Multiply(x=w2763, y=-1.0) -> (x*y=w2765:dbl)
                    n838 = local read "Zoom"() -> (w2798:sgl)
                    n839 = property on="XY Graph 2" class="XYGraph (strict)"("X Scale.Range:Maximum"=w2790, "X Scale.Range:Minimum"=w2789, "Y Scale.Range:Maximum"=w2790, "Y Scale.Range:Minimum"=w2789) -> ()  [unwired: 2 in, 2 out]
                    n840 = Bundle("PointsCoordinates"=w2788, "PointsCoordinates"=w2786) -> (→"Histogram1" →"Histogram2":T16)  [unwired: 1 in]
                    n841 = Subtract(x=w2765, y=360.0) -> (x-y=w2762:dbl)
                    n842 = Divide(x=w2760, y=w2798) -> (x/y=w2759:dbl[][])
                    n843 = Reciprocal(x=w2743) -> (1/x=w2742:dbl)
                    n844 = Divide(x=w2762, y=360.0) -> (x/y=w2840:dbl)
                    n845 = Multiply(x=w2752, y=w2751) -> ()  [unwired: 1 out]
                    n846 = local write "X-pixels FreeLine"(w2745) -> ()
                    n847 = Multiply(x=w2840, y=6.283185307179586) -> (x*y=w2838:dbl)
                    n848 = Multiply(x=w2742, y=sgl 1000000.0) -> (x*y=→"pixel dwell time [us] FreeLine":dbl)
                    n849 = Sine(x=w2838) -> (sin(x)=w2834:dbl)
                    n850 = Cosine(x=w2838) -> (cos(x)=w2833:dbl)
                    n851 = local read "x jog"() -> (w2794:sgl)
                    n852 = Array Subset(array=w2768, index=0, length=1) -> (w2826:dbl[])
                    n853 = Array Subset(array=w2767, index=0, length=1) -> (w2825:dbl[])
                    n854 = Negate(x=w2834) -> (-x=w2837:dbl)
                    n855 = local read "y jog"() -> (w2793:sgl)
                    n856 = Bundle("Signal x"=w2768, "Signal y"=w2767) -> (w2824:cluster{"Signal x":dbl[], "Signal y":dbl[]})  [unwired: 1 in]
                    n857 = Bundle(w2826, w2825) -> (w2823:cluster{dbl[], dbl[]})  [unwired: 1 in]
                    n858 = Divide(x=w2743, y=w2745) -> (x/y=w2744:dbl)
                    n859 = Build Array(w2833, w2837) -> (w2836:dbl[])
                    n860 = Build Array(w2834, w2833) -> (w2835:dbl[])
                    n861 = Decrement(x=w2745) -> (x-1=w2819:i32)
                    n862 = local write "z frequency"(w2744) -> ()
                    n863 = Build Array(w2836, w2835) -> (w2761:dbl[][])
                    n864 = Initialize Array(w2751, w2749) -> (w2750:sgl[])
                    n865 = Array Subset(array=w2768, index=w2819, length=w2820) -> (w2821:dbl[])
                    n866 = Array Subset(array=w2767, index=w2819, length=w2820) -> (w2822:dbl[])
                    n867 = call-poly <vilib>:"A x B.vi"("B"=w2759, "A"=w2761) -> ("A x B"=w2758:T15)  [unwired: 1 out]
                    n868 = Index Array(array=w2758, index (row)=0 ("disabled index (col)")) -> (element=w2797:dbl[])  [unwired: 1 in]
                    n869 = Index Array(array=w2758, index (row)=1 ("disabled index (col)")) -> (element=w2796:dbl[])  [unwired: 1 in]
                    n870 = Add(x=w2796, y=w2793) -> (x+y=w2795:dbl[])
                    n871 = Add(x=w2797, y=w2794) -> (x+y=w2774:dbl[])
                    n872 = Build Array(w2774, w2795) -> (w2753:dbl[][])
                    n873 = local write "ScanLineFreeLine"(w2753) -> ()
                    n874 = Bundle(w2821, w2822) -> (w2818:cluster{dbl[], dbl[]})  [unwired: 1 in]
                    n875 = Build Array (concatenate)(w2753, w2755, w2750) -> (w2754:dbl[][])
                    n876 = Build Array(w2824, w2823, w2818) -> (w2814:cluster{"Signal x":dbl[], "Signal y":dbl[]}[])
                    n877 = local write "XY Graph 1"(w2814) -> ()
                    n878 = local write "XY Graph 2"(w2814) -> ()
                  }
                }
                n879 = Bundle("sample mode"=w2685, "sample mode"=w2685) -> (w2684:cluster{"sample mode":i32, "sample mode":i32})  [unwired: 1 in]
                n880 = Concatenate Strings(w2688, tag "/ao0," ("physical channels"), w2688, tag "/ao1," ("physical channels"), w2688, tag "/ao2," ("physical channels"), w2688, tag "/ao3" ("physical channels")) -> (w2690:string)
                n881 = Type Cast(type=w2687, x=w2690) -> (*(type *) &x=w2686:tag)
              }
            }
          }
          frame True {
            n882 = case shown="True" "NewScanpattern" {
              tunnel: [w2932 w2942] -> w2852
              tunnel: [w2924 w2933] -> w2850
              tunnel: [w2925 w2934] -> w2849
              tunnel: [w2930 w2939] -> w2848
              tunnel: [w2924 w2933] -> w2845
              frame False {
                n883 = local read "ParametersFScope"() -> (w2931:T7)
                n884 = local read "ScanLineFScope"() -> (w2932:sgl[][])
                n885 = Unbundle(w2931) -> ("X frequeny [Hz]"=w2926:i32, "Y frequency \n[Hz]"=w2930:i32, "frequeny Trim"=w2927:dbl, "Samples/s"=w2924:i32)  [unwired: 2 out]
                n886 = local write "Pixel Clock (Hz) FScope"(w2924) -> ()
                n887 = Divide(x=w2927, y=200.0) -> (x/y=w2928:dbl)
                n888 = Add(x=w2926, y=w2928) -> (x+y=w2925:dbl)
              }
              frame True {
                n889 = call "LissajousPatternFScope.vi"("f max Y [Hz]"="f max Y", "f min Y [Hz]"="f min Y", "f max X [Hz]"="f max X", "f min X [Hz]"="f min X") -> ("Parameters"=w2940:T7, "ScanData"=w2942:dbl[][])  [unwired: 1 out]
                "ScanLineFScope" <- w2942
                "ParametersFScope" <- w2940
                n890 = Unbundle(w2940) -> ("X frequeny [Hz]"=w2935:i32, "Y frequency \n[Hz]"=w2939:i32, "frequeny Trim"=w2936:dbl, "Samples/s"=w2933:i32)  [unwired: 2 out]
                "Pixel Clock (Hz) FScope" <- w2933
                n891 = local write "NewScanpattern"(FALSE ("NewScanpattern")) -> ()
                n892 = Divide(x=w2936, y=200.0) -> (x/y=w2938:dbl)
                n893 = Add(x=w2935, y=w2938) -> (x+y=w2934:dbl)
              }
            }
            n894 = local read "scans to read"() -> (w2847:sgl)
            n895 = Reciprocal(x=w2845) -> (1/x=w2846:dbl)
            n896 = Multiply(x=w2846, y=w2847) -> (x*y=w2844:dbl)
            n897 = Reciprocal(x=w2844) -> (1/x=w2843:dbl)
            n898 = local write "Frame rate [Hz]"(w2843) -> ()
            n899 = case shown="2" w2853 {
              tunnel: [w2876 w2894 w2913] -> w2862
              tunnel: w2852 -> [w2874 w2892 w2912]
              tunnel: [w2867 w2885 w2907] -> w2855
              tunnel: [w2866 w2884 w2906] -> w2854
              tunnel: "LS X/Y" -> [_ _ w2905]
              tunnel: w2850 -> [_ _ w2900]
              tunnel: w2849 -> [_ _ w2898]
              tunnel: w2848 -> [_ _ w2899]
              frame 0, Default {
                w2865 = 10123 items=["Finite Samples"=10178, "Continuous Samples"=10123, "Hardware Timed Single Point"=12522] ("sample mode")
                n900 = Index Array(array=w2874, index (row)=0) -> (element=w2873:dbl[])  [unwired: 1 in]
                n901 = Index Array(array=w2874, index (row)=1) -> (element=w2868:dbl[])  [unwired: 1 in]
                n902 = Add(x=w2873, y=w2868) -> (x+y=w2875:dbl[])
                n903 = Array Max & Min(array=w2873) -> (max value=w2871:dbl, min value=w2872:dbl)  [unwired: 2 out]
                n904 = Array Max & Min(array=w2868) -> (max value=w2869:dbl, min value=w2870:dbl)  [unwired: 2 out]
                n905 = Build Array(w2875) -> (w2876:dbl[][])
                n906 = Array Size(array=w2875) -> (size(s)=w2867:i32)
                n907 = global write "GlobelFSCOPE.vi" "X max"(w2871) -> ()
                n908 = global write "GlobelFSCOPE.vi" "X min"(w2872) -> ()
                n909 = global write "GlobelFSCOPE.vi" "Y max"(w2869) -> ()
                n910 = global write "GlobelFSCOPE.vi" "Y min"(w2870) -> ()
                n911 = Bundle("sample mode"=w2865, "sample mode"=w2865) -> (w2866:cluster{"sample mode":i32, "sample mode":i32})  [unwired: 1 in]
              }
              frame 1 {
                w2879 = 10178 items=["Finite Samples"=10178, "Continuous Samples"=10123, "Hardware Timed Single Point"=12522] ("sample mode")
                n912 = Index Array(array=w2892, index (row)=0) -> (element=w2891:dbl[])  [unwired: 1 in]
                n913 = Index Array(array=w2892, index (row)=1) -> (element=w2886:dbl[])  [unwired: 1 in]
                n914 = Add(x=w2891, y=w2886) -> (x+y=w2893:dbl[])
                n915 = Array Max & Min(array=w2891) -> (max value=w2889:dbl, min value=w2890:dbl)  [unwired: 2 out]
                n916 = Array Max & Min(array=w2886) -> (max value=w2887:dbl, min value=w2888:dbl)  [unwired: 2 out]
                n917 = Build Array(w2893) -> (w2894:dbl[][])
                n918 = Array Size(array=w2893) -> (size(s)=w2885:i32)
                n919 = global write "GlobelFSCOPE.vi" "X max"(w2889) -> ()
                n920 = global write "GlobelFSCOPE.vi" "X min"(w2890) -> ()
                n921 = global write "GlobelFSCOPE.vi" "Y max"(w2887) -> ()
                n922 = global write "GlobelFSCOPE.vi" "Y min"(w2888) -> ()
                n923 = local read "Number of Frames"() -> (w2881:sgl)
                n924 = local read "scans to read"() -> (w2883:sgl)
                n925 = local read "Averaging"() -> (w2882:sgl)
                n926 = Compound Arithmetic op=MULTIPLY(w2883, w2882, w2881) -> (w2880:sgl)
                n927 = Bundle(w2880, "sample mode"=w2879) -> (w2884:cluster{sgl, "sample mode":i32})  [unwired: 1 in]
              }
              frame 2 {
                w2901 = 10123 items=["Finite Samples"=10178, "Continuous Samples"=10123, "Hardware Timed Single Point"=12522] ("sample mode")
                n928 = Index Array(array=w2912, index (row)=0) -> (element=w2904:dbl[])  [unwired: 1 in]
                n929 = Index Array(array=w2912, index (row)=1) -> (element=w2902:dbl[])  [unwired: 1 in]
                n930 = Array Max & Min(array=w2904) -> (max value=w2910:dbl, min value=w2911:dbl)  [unwired: 2 out]
                n931 = Array Max & Min(array=w2902) -> (max value=w2908:dbl, min value=w2909:dbl)  [unwired: 2 out]
                n932 = case shown="False" w2905 {
                  tunnel: [w2919 w2923] -> w2903
                  tunnel: w2904 -> [_ w2923]
                  tunnel: w2902 -> [w2919 _]
                  tunnel: w2900 -> [w2918 w2922]
                  tunnel: w2899 -> [w2917 _]
                  tunnel: w2898 -> [_ w2921]
                  tunnel: [w2916 w2920] -> w2897
                  frame False {
                    n933 = Divide(x=w2918, y=w2917) -> (x/y=w2916:dbl)
                  }
                  frame True {
                    n934 = Divide(x=w2922, y=w2921) -> (x/y=w2920:dbl)
                  }
                }
                n935 = global write "GlobelFSCOPE.vi" "X max"(w2910) -> ()
                n936 = global write "GlobelFSCOPE.vi" "X min"(w2911) -> ()
                n937 = global write "GlobelFSCOPE.vi" "Y max"(w2908) -> ()
                n938 = global write "GlobelFSCOPE.vi" "Y min"(w2909) -> ()
                n939 = local write "scans to read"(w2897) -> ()
                n940 = Build Array(w2903) -> (w2913:dbl[][])
                n941 = Array Size(array=w2903) -> (size(s)=w2907:i32)
                n942 = Bundle("sample mode"=w2901, "sample mode"=w2901) -> (w2906:cluster{"sample mode":i32, "sample mode":i32})  [unwired: 1 in]
              }
            }
            "Scanlength" <- w2855
            n943 = Concatenate Strings(w2857, tag "/ao0" ("physical channels")) -> (w2861:string)
            n944 = Type Cast(type=w2858, x=w2861) -> (*(type *) &x=w2859:tag)
          }
        }
        "ScanSignals" <- w2004
        n945 = Subtract(x=w1878, y=2.0) -> (x-y=w1880:dbl)
        n946 = case shown="True" "Stimulus" {
          tunnel: w1878 -> [_ w2068]
          tunnel: [u32 2 ("low ticks") w2067] -> w1883
          tunnel: [w2061 w2066] -> w1882
          tunnel: [0.0 w2065] -> w1881
          tunnel: w1880 -> [w2061 _]
          tunnel: w1855 -> [_ w2064]
          frame False {
          }
          frame True {
            n947 = Multiply(x="Stimulus Duration [s]", y=sgl 1000000.0) -> (x*y=w2070:sgl)
            n948 = Divide(x=w2070, y=w2064) -> (x/y=w2067:sgl)
            n949 = Multiply(x="Interval [x Lines]", y=w2068) -> (x*y=w2065:dbl)
            n950 = Subtract(x=w2065, y=w2067) -> (x-y=w2066:dbl)
          }
        }
        n951 = call-poly <vilib>:"DAQmx Create Channel (CO-Pulse Generation-Ticks).vi"("high ticks"=w1883, "low ticks"=w1882, "counter"=w1925, "source of ticks"=w1937, "error in"=w1921, "initial delay"=w1881) -> ("task out"=w2021:refnum<k21>, "error out"=w2020:errorcluster)  [unwired: 8 in]
        n952 = property on="Linescan mode" class="Bool (strict)"("Visible"=w1860) -> ()  [unwired: 2 in, 2 out]
        n953 = call-poly <vilib>:"DAQmx Timing (Implicit).vi"("task/channels in"=w2021, "sample mode"=w2019, "error in"=w2020) -> ("task out"=w2018:refnum<k21>, "error out"=w2017:errorcluster)  [unwired: 11 in]
        n954 = Greater Or Equal?(x=w1918, y=u16 1) -> (x >= y?=w1916:bool)
        n955 = call <vilib>:"DAQmx Start Task.vi"("task/channels in"=w2018, "error in"=w2017) -> ("task out"=w1962:refnum<k21>, "error out"=w1923:errorcluster)  [unwired: 12 in]
        n956 = local read "Scangraph scaling"() -> (w1851:sgl)
        n957 = local read "frame/line indicator"() -> (w1920:u16)
        n958 = Multiply(x=w1952, y=w1878) -> (x*y=w1953:dbl)
        n959 = local read "AO/DIO Device"() -> (w1964:tag)
        n960 = local read "Fiberscope\nMode"() -> (w1892:bool)
        n961 = property on="XScale" class="Bool (strict)"("Visible"=w1861) -> ()  [unwired: 2 in, 2 out]
        n962 = property on="Test Run?" class="Bool (strict)"("Visible"=w1861) -> ()  [unwired: 2 in, 2 out]
        n963 = property on="Scale" class="DigNum (strict)"("Visible"=w1861) -> ()  [unwired: 2 in, 2 out]
        n964 = property on="Int Corr?" class="Bool (strict)"("Visible"=w1861) -> ()  [unwired: 2 in, 2 out]
        n965 = Subtract(x=w1953, y=2.0) -> (x-y=w1875:dbl)
        n966 = case shown="True" "Case Constant\n(See Context Help)" {
          tunnel: w1878 -> [_ w2056]
          tunnel: [u32 2 ("low ticks") w2055] -> w1876
          tunnel: [w2049 w2054] -> w1874
          tunnel: [0.0 w2053] -> w1877
          tunnel: w1875 -> [w2049 _]
          tunnel: w1855 -> [_ w2052]
          frame False {
          }
          frame True {
            n967 = Multiply(x="Stimulus Duration [s] 2", y=sgl 1000000.0) -> (x*y=w2058:sgl)
            n968 = Divide(x=w2058, y=w2052) -> (x/y=w2055:sgl)
            n969 = Multiply(x="Interval [x Lines] 2", y=w2056) -> (x*y=w2053:dbl)
            n970 = Subtract(x=w2053, y=w2055) -> (x-y=w2054:dbl)
          }
        }
        n971 = Array Subset(array=w2004, length (row)=2 ("length")) -> (w2003:dbl[][])  [unwired: 3 in]
        n972 = local read "AO/DIO Device"() -> (w1927:tag)
        n973 = Concatenate Strings(w1964, tag "/port0" ("lines")) -> (w1972:string)
        n974 = Array Max & Min(array=w2003) -> (max value=w2006:dbl, min value=w2005:dbl)  [unwired: 2 out]
        n975 = local read "AO/DIO Device"() -> (w1933:tag)
        n976 = Decrement(x=w1851) -> (x-1=w1853:sgl)
        n977 = Equal To 0?(x=w1920) -> (x = 0?=w1919:bool)
        n978 = case shown="True" w1892 {
          tunnel: [w2074 w2077] -> w2026
          tunnel: w1919 -> [w2073 _]
          frame False {
            n979 = case shown="False" w2073 {
              tunnel: [w2075 w2076] -> w2074
              frame False {
                w2075 = 10097 items=["Allow Regeneration"=10097, "Do Not Allow Regeneration"=10158] ("RegenMode")
              }
              frame True {
                w2076 = 10158 items=["Allow Regeneration"=10097, "Do Not Allow Regeneration"=10158] ("RegenMode")
              }
            }
          }
          frame True {
            w2077 = 10097 items=["Allow Regeneration"=10097, "Do Not Allow Regeneration"=10158] ("RegenMode")
          }
        }
        n980 = Type Cast(type=tag "" ("lines"), x=w1972) -> (*(type *) &x=w1969:tag)
        n981 = Negate(x=w1853) -> (-x=w1854:sgl)
        n982 = Negate(x=w1851) -> (-x=w1852:sgl)
        n983 = In Range and Coerce(upper limit=10.0 ("y"), x=w1887, lower limit=-10.0 ("y")) -> (coerced(x)=w1888:dbl[][])  [unwired: 1 out]
        n984 = local read "AO/DIO Device"() -> (w1912:tag)
        n985 = Concatenate Strings(tag "/" ("destination terminal"), w1912) -> (w1906:string)
        n986 = Concatenate Strings(tag "/" ("destination terminal"), w1927, tag "/ao/SampleClock" ("source of ticks")) -> (w1932:string)
        n987 = call-poly <vilib>:"DAQmx Create Channel (DI-Digital Input).vi"("lines"=w1969, "error in"=w1921) -> ("task out"=w1951:refnum<k21>, "error out"=w1949:errorcluster)  [unwired: 12 in]
        n988 = Index Array(array=w2003, index (row)=1 ("index")) -> (element=w2040:dbl[])  [unwired: 1 in]
        n989 = Concatenate Strings(w1933, tag "/ctr1" ("counter")) -> (w1935:string)
        n990 = Concatenate Strings(tag "/" ("destination terminal"), w1964, tag "/ao/SampleClock" ("source terminal")) -> (w1968:string)
        n991 = Greater?(x=w2006, y=w1853) -> (0:w2044:bool)
        n992 = Less?(x=w2005, y=w1854) -> (x < y?=w2045:bool)
        n993 = Type Cast(type=tag "" ("source of ticks"), x=w1932) -> (*(type *) &x=w1928:tag)
        n994 = Or(x=w2044, y=w2045) -> (x .or. y?=w2042:bool)
        n995 = Index Array(array=w2003, index (row)=0 ("index")) -> (element=w2039:dbl[])  [unwired: 1 in]
        n996 = Type Cast(type=tag "" ("counter"), x=w1935) -> (*(type *) &x=w1934:tag)
        n997 = Type Cast(type=tag "" ("source terminal"), x=w1968) -> (*(type *) &x=w1963:tag)
        n998 = Concatenate Strings(tag "/" ("destination terminal"), w1912) -> (w1896:string)
        n999 = case shown="True" w2042 {
          tunnel: [u32 0 w3029] -> w2041
          tunnel: w2003 -> [_ w3024]
          tunnel: w1852 -> [_ w3022]
          tunnel: w1851 -> [_ w3021]
          frame False {
          }
          frame True {
